vi "Ejercicio 2.1.vi"() -> ()   [LabVIEW 2020]
panel:
  out "Resultados Arreglo":i32[](array[numeric])
  out "Resultado":i64
  in  "Limite de valores en el arreglo":i32
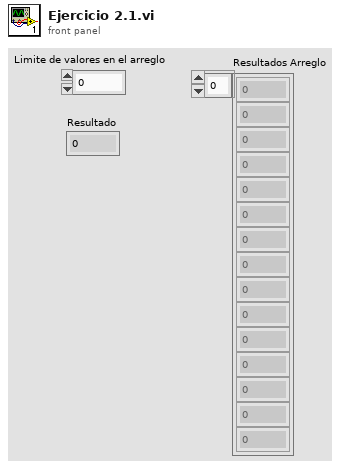
[diagram p1: front panel]
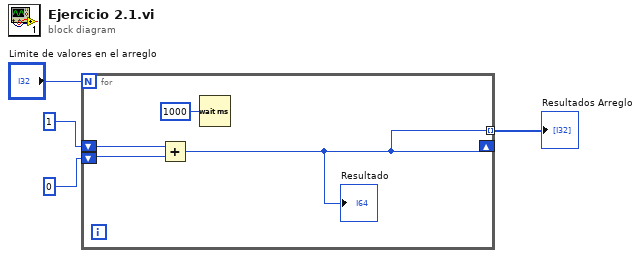
[diagram p0: block diagram]
diagram:
  n1 = for {
    N: "Limite de valores en el arreglo" -> [_]
    shift-right: [w5] -> _
    shift-left: 1 -> [w8]
    shift-left: 0 -> [w7]
    tunnel: [w5] -> w1 mode=indexing
    n2 = Add(x=w8, y=w7) -> (x+y=w5:i32)
    "Resultado" <- w5
    n3 = Wait (ms)(milliseconds to wait=u32 1000) -> ()  [unwired: 1 out]
  }
  "Resultados Arreglo" <- w1
